vi "ACCUMULATE.vi"(6 "Reset?":bool, 9 "Input":dbl, 10 "Enabled?":bool=TRUE) -> (2 "Accumulation":dbl)   [LabVIEW 2015]
doc: "While enabled, each iteration that Enabled is true, Input will be added to Accumulation.\nEach iteration that Enabled is false, Input will be ignored.\nWhen Reset is true, Accumualtion will be set to zero."
uses:
  <vilib>/functionblocks/Accumulate/Accumulate/Accumulate.vi
  <vilib>/functionblocks/FB Core/FB Core.xnode
  <vilib>/functionblocks/NI_FunctionBlock Libraries.lvlib
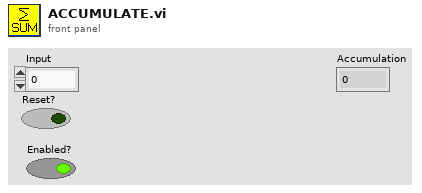
[diagram p1: front panel]
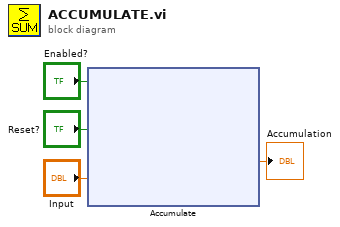
[diagram p0: block diagram]
diagram:
  n1 = xnode "Accumulate"("reset"="Reset?", "input"="Input", "enable"="Enabled?") -> ("accumulation"=→"Accumulation":dbl)  [unwired: 1 in, 1 out]
